vi "CarMain_SENSOR_CONTROL_v2.vi"() -> ()   [LabVIEW 2013]
panel:
  out "Right PR Black":bool
  out "Mid PR Black":bool
  out "Left PR Black":bool
  out "Right PR Voltage 3":dynamicdata(graph)
  out "Right PR (volts) 3":dbl
  out "Mid PR Voltage 2":dynamicdata(graph)
  out "Mid PR (volts) 2":dbl
  out "Left PR Voltage":dynamicdata(graph)
  out "Right IR Voltage":dynamicdata(graph)
  out "Mid IR Voltage":dynamicdata(graph)
  out "Left IR Voltage":dynamicdata(graph)
  out "Left PR (volts)":dbl
  out "Voltage 3":dbl
  out "Right IR":bool
  out "Voltage 2":dbl
  out "Middle IR":bool
  out "Left IR":bool
  out "Voltage":dbl
  in  "stop":bool
  in  "Stop Array":bool[](array[boolean]) caption="Stop"
  in  "Forward Array":bool[](array[boolean]) caption="Forward"
  in  "Backward Array":bool[](array[boolean]) caption="Backward"
  in  "Turn Left Array":bool[](array[boolean]) caption="Turn Left"
  in  "Turn Right Array":bool[](array[boolean]) caption="Turn Right"
  # "NOTE: This is the final VI for your project. \nWhat you need to do is complete this template by\nadding the boolean (digital) logic on the back panel.\n(See block diagram)"
  # "Indicates if comparison on block diagram is true."
  # "Set your array values. For a value of 1, \nclick on the dot and make it turn black.\nFor a value of zero, leave the dot light gray"
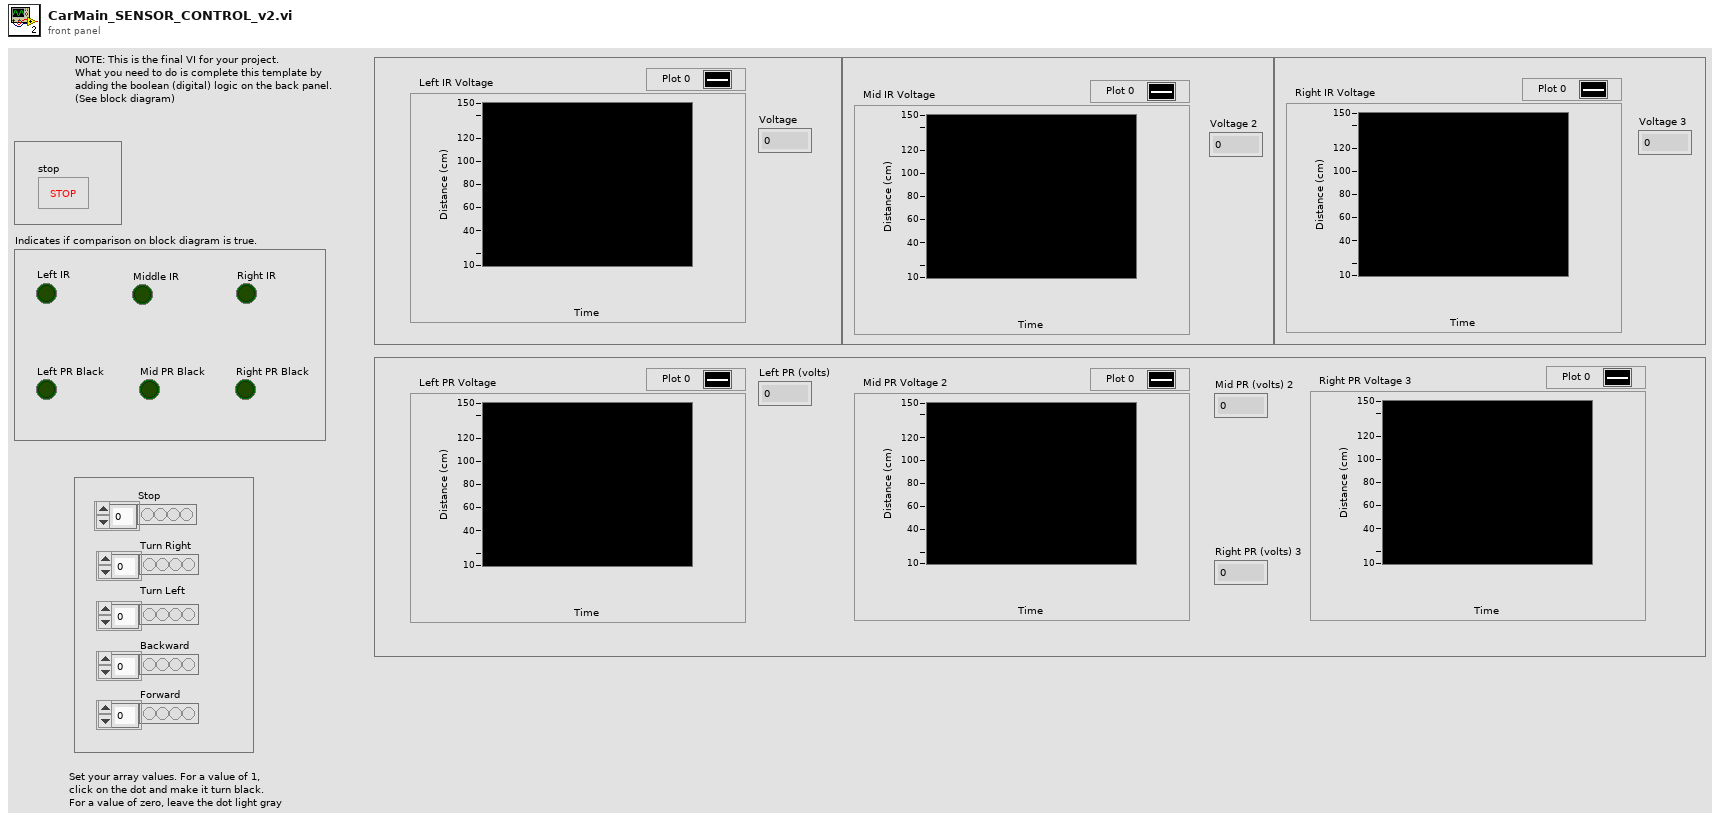
[diagram p1: front panel]
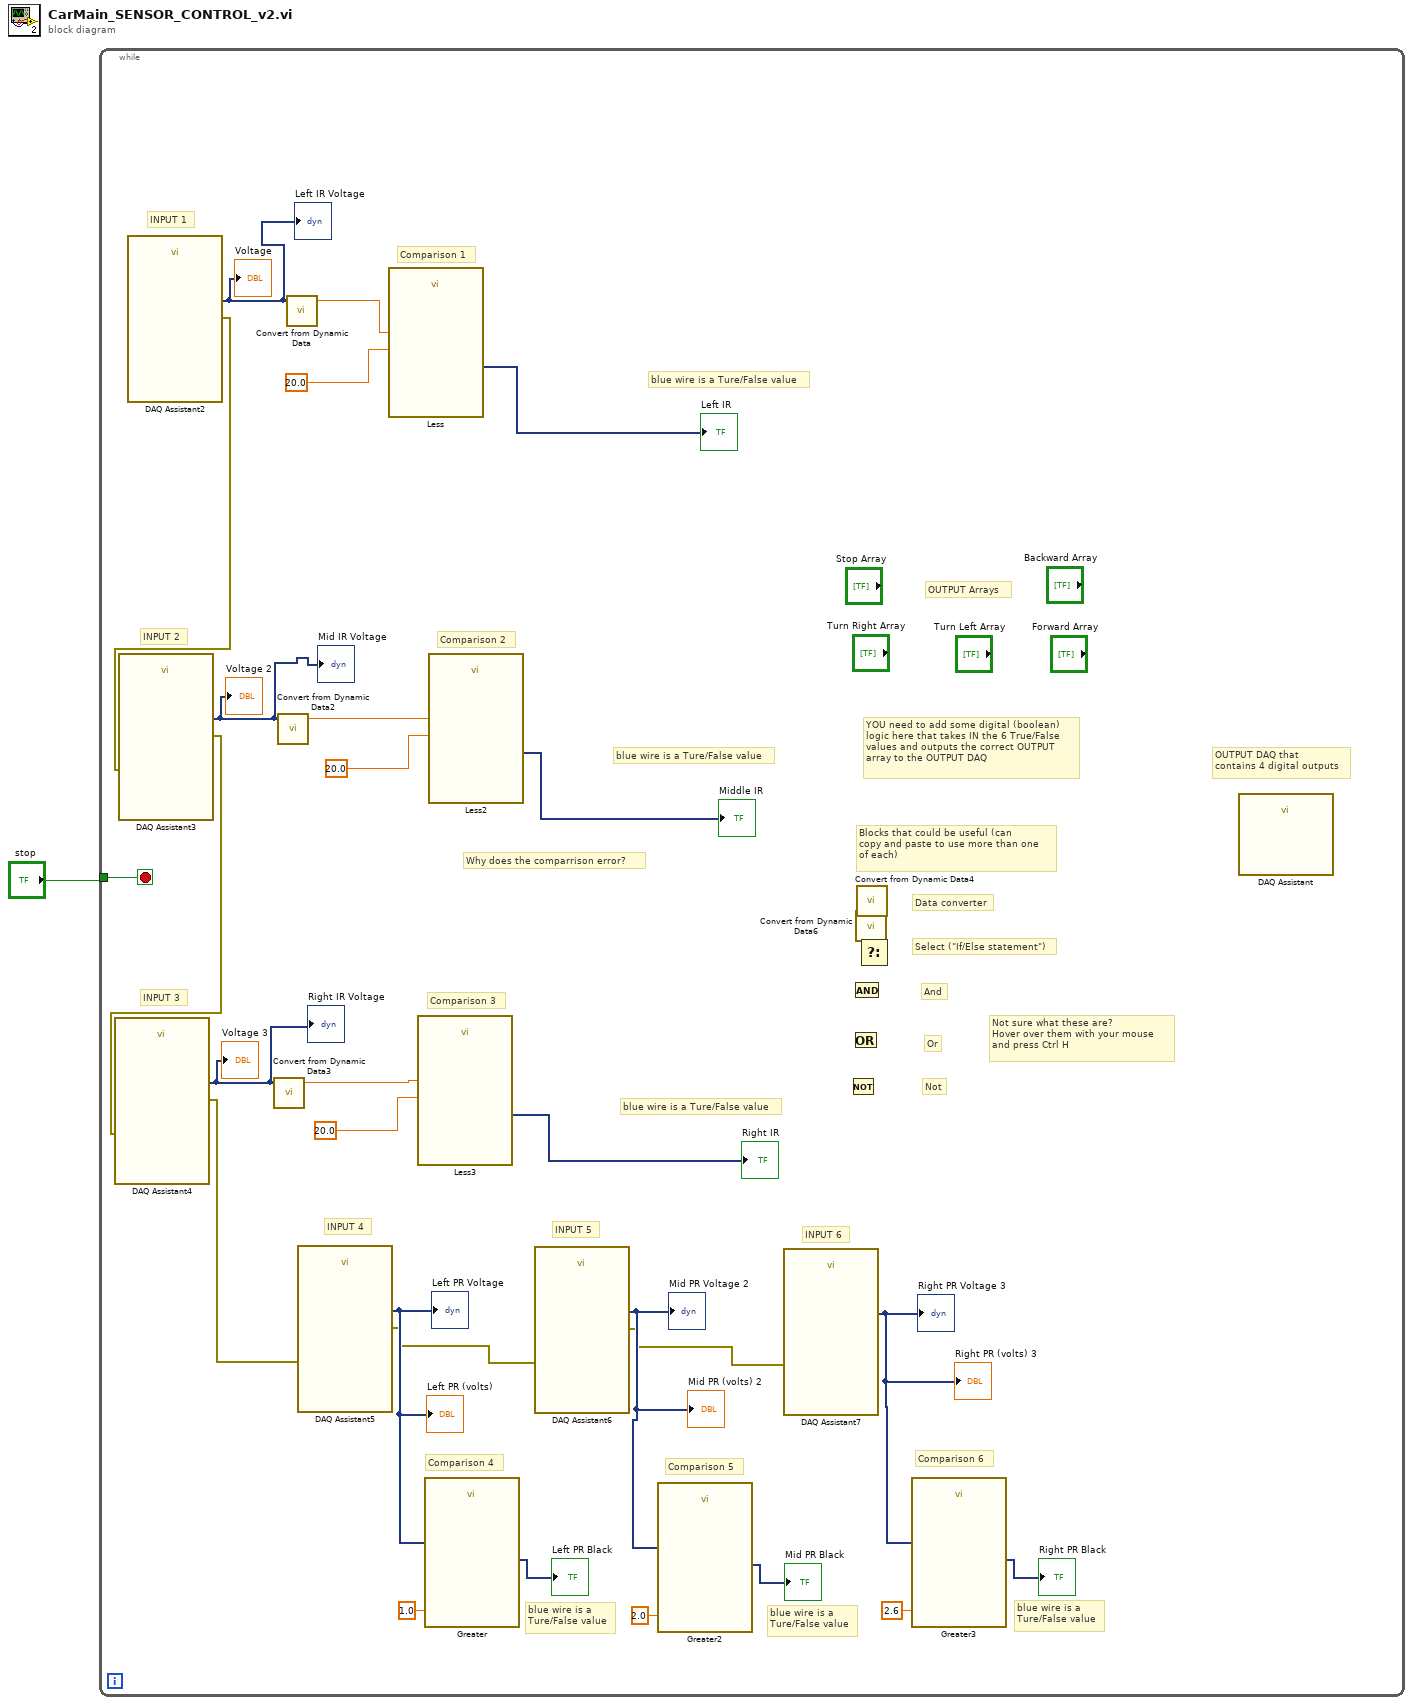
[diagram p0: block diagram]
diagram:
  n1 = while {
    tunnel: "stop" -> [w28]
    stop <- w28 stop-if-true
    # "Why does the comparrison error?"
    # "Not sure what these are? \nHover over them with your mouse\nand press Ctrl H"
    # "Not"
    # "Or"
    # "And"
    # "Select (\"If/Else statement\")"
    # "Data converter"
    # "Blocks that could be useful (can \ncopy and paste to use more than one\nof each)"
    # "YOU need to add some digital (boolean)\nlogic here that takes IN the 6 True/False \nvalues and outputs the correct OUTPUT \narray to the OUTPUT DAQ"
    # "blue wire is a \nTure/False value"
    # "blue wire is a\nTure/False value"
    # "blue wire is a \nTure/False value"
    # "blue wire is a Ture/False value"
    # "blue wire is a Ture/False value"
    # "blue wire is a Ture/False value"
    # "OUTPUT DAQ that\ncontains 4 digital outputs"
    # "OUTPUT Arrays"
    # "Comparison 6"
    # "INPUT 6"
    # "Comparison 5"
    # "INPUT 5"
    # "Comparison 4"
    # "INPUT 4"
    # "Comparison 3"
    # "INPUT 3"
    # "Comparison 2"
    # "Comparison 1"
    # "INPUT 2"
    # "INPUT 1"
    n2 = call "DAQ Assistant2"() -> ("data"=w21:dynamicdata, "error out"=w27:errorcluster)  [unwired: 17 in, 1 out]
    "Voltage" <- w21
    "Left IR Voltage" <- w21
    n3 = call "DAQ Assistant3"("error in"=w27) -> ("data"=w20:dynamicdata, "error out"=w26:errorcluster)  [unwired: 16 in, 1 out]
    "Voltage 2" <- w20
    "Mid IR Voltage" <- w20
    n4 = call "DAQ Assistant4"("error in"=w26) -> ("data"=w19:dynamicdata, "error out"=w7:errorcluster)  [unwired: 16 in, 1 out]
    "Voltage 3" <- w19
    "Right IR Voltage" <- w19
    n5 = call "Convert from Dynamic Data3"("Dynamic Data Type"=w19) -> ("Scalar"=w4:dbl)  [unwired: 3 in]
    n6 = call "Convert from Dynamic Data2"("Dynamic Data Type"=w20) -> ("Scalar"=w5:dbl)  [unwired: 3 in]
    n7 = call "Convert from Dynamic Data"("Dynamic Data Type"=w21) -> ("Scalar"=w6:dbl)  [unwired: 3 in]
    n8 = call "DAQ Assistant5"("error in"=w7) -> ("data"=w10:dynamicdata, "error out"=w8:errorcluster)  [unwired: 16 in, 1 out]
    "Left PR (volts)" <- w10
    "Left PR Voltage" <- w10
    n9 = call "Less"("Constant Value to Compare Against"=20.0, "Operand 1"=w6) -> ("Result"=→"Left IR":dynamicdata)  [unwired: 8 in, 1 out]
    n10 = call "Less3"("Constant Value to Compare Against"=20.0, "Operand 1"=w4) -> ("Result"=→"Right IR":dynamicdata)  [unwired: 8 in, 1 out]
    n11 = call "Greater"("Constant Value to Compare Against"=1.0, "Operand 1"=w10) -> ("Result"=→"Left PR Black":dynamicdata)  [unwired: 8 in, 1 out]
    n12 = call "Less2"("Constant Value to Compare Against"=20.0, "Operand 1"=w5) -> ("Result"=→"Middle IR":dynamicdata)  [unwired: 8 in, 1 out]
    n13 = call "DAQ Assistant6"("error in"=w8) -> ("data"=w17:dynamicdata, "error out"=w9:errorcluster)  [unwired: 16 in, 1 out]
    "Mid PR (volts) 2" <- w17
    "Mid PR Voltage 2" <- w17
    n14 = call "Greater2"("Constant Value to Compare Against"=2.0, "Operand 1"=w17) -> ("Result"=→"Mid PR Black":dynamicdata)  [unwired: 8 in, 1 out]
    n15 = call "DAQ Assistant7"("error in"=w9) -> ("data"=w18:dynamicdata)  [unwired: 16 in, 2 out]
    "Right PR (volts) 3" <- w18
    "Right PR Voltage 3" <- w18
    n16 = Not() -> ()  [unwired: 1 in, 1 out]
    n17 = Or() -> ()  [unwired: 2 in, 1 out]
    n18 = And() -> ()  [unwired: 2 in, 1 out]
    n19 = call "Convert from Dynamic Data6"() -> ()  [unwired: 4 in, 1 out]
    n20 = call "Convert from Dynamic Data4"() -> ()  [unwired: 4 in, 1 out]
    n21 = Select() -> ()  [unwired: 3 in, 1 out]
    n22 = call "Greater3"("Constant Value to Compare Against"=2.6, "Operand 1"=w18) -> ("Result"=→"Right PR Black":dynamicdata)  [unwired: 8 in, 1 out]
    n23 = call "DAQ Assistant"() -> ()  [unwired: 18 in, 2 out]
  }
